vi "Destroy DSF Configuration Session.vi"(8 "error in (no error)":errorcluster, 11 "DSF Configuration Session in":T1) -> (0 "error out":errorcluster)   [LabVIEW 2017]
uses:
  Controls/Session/DSF Configuration Reference.ctl
  Controls/DSF File Format/Internal.DSF Configuration.ctl
  Public/Controls/DSF Version Info.ctl
  Controls/DSF File Format/Internal.DSF Plugin with ID.ctl
  Controls/DSF File Format/Internal.DSF Plugin Info.ctl
  Public/Controls/DSF Timing Info.ctl
  Controls/DSF File Format/Internal.DSF Group with ID.ctl
  Controls/DSF File Format/Internal.DSF Group Info.ctl
  Controls/DSF File Format/Internal.DSF Transfer with ID.ctl
  Controls/DSF File Format/Internal.DSF Transfer Info.ctl
  Controls/DSF File Format/Internal.DSF Channel with ID.ctl
  Controls/DSF File Format/Internal.DSF Channel Info.ctl
  Controls/DSF File Format/Internal.DSF Settings with ID.ctl
  Controls/DSF File Format/Internal.DSF Settings Info.ctl
  DSF Core.lvlib
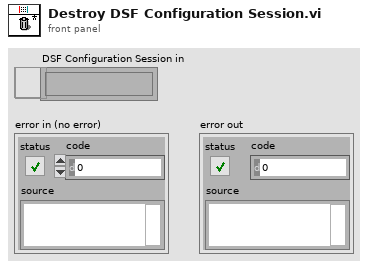
[diagram p1: front panel]
types:
  T1 = typedef "DSF Configuration Reference.ctl" = refnum<data-value>
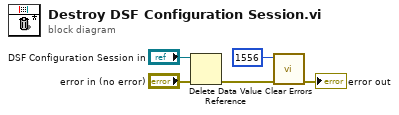
[diagram p0: block diagram]
diagram:
  n1 = Delete Data Value Reference(data value reference="DSF Configuration Session in", error in="error in (no error)") -> (error out=w5:errorcluster)  [unwired: 1 out]
  n2 = call <vilib>:"Clear Errors.vi"("error in (no error)"=w5, "specific error code to clear (0: all)"=1556) -> ("error out"=→"error out":errorcluster)  [unwired: 4 in, 1 out]
